vi "one shot error.vi"(11 "error in":errorcluster) -> ()   [LabVIEW 2013, in "NISE_CEF_TreeControl.lvlib"]
uses:
  NISE_CEF_TreeControl.lvlib
  <vilib>/Utility/error.llb/DialogType.ctl
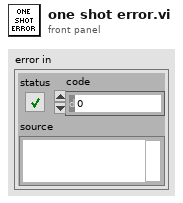
[diagram p1: front panel]
types:
  T1 = typedef "DialogType.ctl" = u16
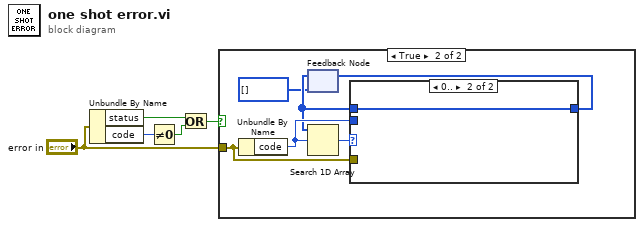
[diagram p0: block diagram]
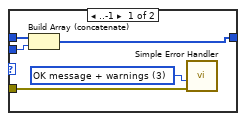
[diagram p3: hidden frame]
diagram:
  n1 = Unbundle By Name("error in") -> ("status"=w3:bool, "code"=w5:i32)
  n2 = Not Equal To 0?(x=w5) -> (x != 0?=w4:bool)
  n3 = Or(x=w3, y=w4) -> (x .or. y?=w2:bool)
  n4 = case shown="True" w2 {
    tunnel: "error in" -> [_ w10]
    frame False {
    }
    frame True {
      n5 = Unbundle By Name(w10) -> ("code"=w9:i32)
      n6 = feedback #1(i32[] []) -> (w7:i32[])
      n7 = Search 1D Array(1D array=w7, element=w9) -> (index of element=w11:i32)  [unwired: 1 in]
      n8 = case shown="0.." w11 {
        tunnel: w10 -> [w15 _]
        tunnel: w9 -> [w14 _]
        tunnel: [w13 w17] -> w8
        tunnel: w7 -> [w12 w17]
        frame ..-1 {
          w16 = T1 3 items=["no dialog", "OK message", "continue or stop message", "OK message + warnings", "continue/stop + warnings"] ("type of dialog (OK msg:1)")
          n9 = Build Array (concatenate)(w12, w14) -> (w13:i32[])
          n10 = call <vilib>:"Simple Error Handler.vi"("type of dialog (OK msg:1)"=w16, "error in (no error)"=w15) -> ()  [unwired: 3 in, 5 out]
        }
        frame 0.. {
        }
      }
      n11 = feedback-in #1(w8) -> ()
    }
  }
